vi "run_object.vi"(6 "ms timeout (0:default)":i32, 8 "error in (no error)":errorcluster, 10 "query":string, 11 "rethinkdb in":T1) -> (0 "error out":errorcluster, 2 "response":variant, 3 "rethinkdb out":T1)   [LabVIEW 2017, in "rethinkdb.lvlib"]
uses:
  rethinkdb.lvlib
  refnum.ctl
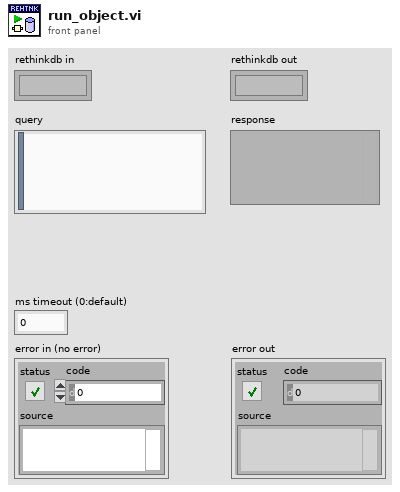
[diagram p1: front panel]
types:
  T1 = typedef "rethinkdb.lvlib/refnum.ctl" = refnum<k1>
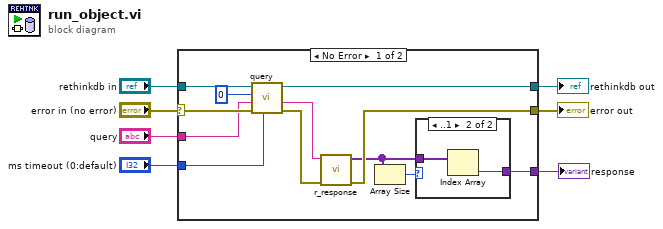
[diagram p0: block diagram]
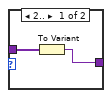
[diagram p2: hidden frame]
diagram:
  n1 = case shown="No Error" "error in (no error)" {
    selector: "error in (no error)" -> [w19 w25]
    tunnel: "ms timeout (0:default)" -> [w18 _]
    tunnel: "query" -> [w17 _]
    tunnel: "rethinkdb in" -> [w16 w24]
    tunnel: [w15 w24] -> w3
    tunnel: [w11 w25] -> w2
    tunnel: [w10 _] -> w1
    frame No Error {
      n2 = call "query.vi"("ms timeout (0:default)"=w18, "error in (no error)"=w19, "query"=w17, "token in (random)"=u64 0, "rethinkdb in"=w16) -> ("error out"=w12:errorcluster, "response"=w13:string, "rethinkdb out"=w15:T1)  [unwired: 3 in, 1 out]
      n3 = call "r_response.vi"("error in (no error)"=w12, "response"=w13) -> ("error out"=w11:errorcluster, "values"=w9:variant[])  [unwired: 8 in]
      n4 = Array Size(array=w9) -> (size(s)=w8:i32)
      n5 = case shown="..1" w8 {
        tunnel: [w20 w23] -> w10
        tunnel: w9 -> [w21 w22]
        frame 2.. {
          n6 = To Variant(anything=w21) -> (Variant=w20:variant)
        }
        frame ..1 {
          n7 = Index Array(array=w22) -> (element=w23:variant)  [unwired: 1 in]
        }
      }
    }
    frame Error {
    }
  }
  "error out" <- w2
  "rethinkdb out" <- w3
  "response" <- w1
